vi "Assignment #3 - Sarah Bailey.vi"() -> ()   [LabVIEW 2013]
panel:
  out "Calculated Tolerance":dbl
  out "ROOT":dbl
  in  "Tolerance":dbl min=0.0
  in  "XHI":dbl=1e-16 min=1e-16
  in  "XLO":dbl=1e-16 min=1e-16
  # "Developed by: Sarah Bailey\nEngineering Applications Lab\nAssignment #3\nProfessor Wellin\nWorked with: Clair Cummingham and Alex Offredi"
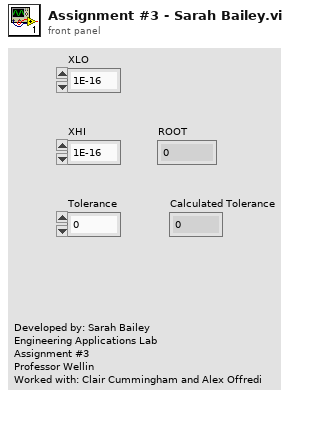
[diagram p1: front panel]
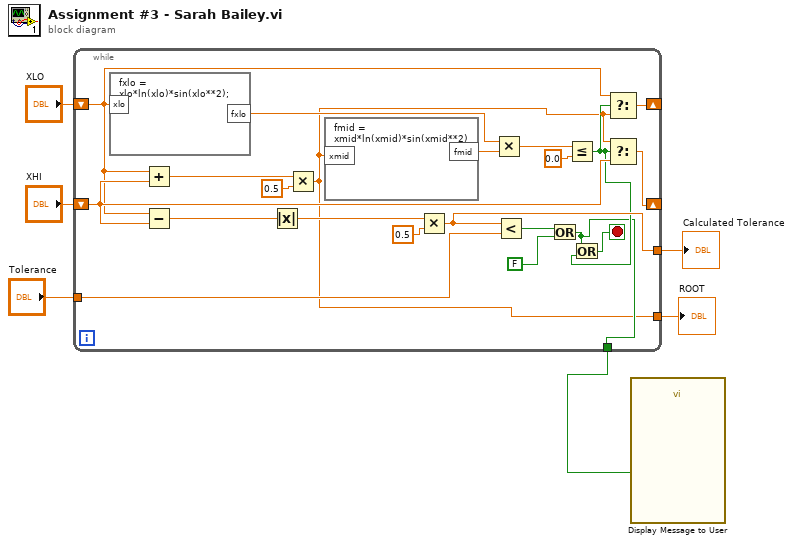
[diagram p0: block diagram]
diagram:
  n1 = while {
    shift-right: [w22] -> _
    shift-left: "XLO" -> [w16]
    shift-right: [w23] -> _
    shift-left: "XHI" -> [w21]
    tunnel: [w7] -> w4
    tunnel: [w8] -> w3
    tunnel: "Tolerance" -> [w12]
    tunnel: [w11] -> w1
    stop <- w9 stop-if-true
    n2 = formula code="fxlo = xlo*ln(xlo)*sin(xlo**2);"("xlo"=w16) -> ("fxlo"=w15:dbl)
    n3 = Add(x=w16, y=w21) -> (x+y=w27:dbl)
    n4 = Subtract(x=w16, y=w21) -> (x-y=w20:dbl)
    n5 = Absolute Value(x=w20) -> (abs(x)=w19:dbl)
    n6 = Multiply(x=w27, y=0.5) -> (x*y=w7:dbl)
    n7 = formula code="fmid = xmid*ln(xmid)*sin(xmid**2) ;"("xmid"=w7) -> ("fmid"=w14:dbl)
    n8 = Multiply(x=w19, y=0.5) -> (x*y=w11:dbl)
    n9 = Multiply(x=w15, y=w14) -> (x*y=w25:dbl)
    n10 = Less?(x=w11, y=w12) -> (x < y?=w17:bool)
    n11 = Or(x=w17, y=FALSE) -> (x .or. y?=w8:bool)
    n12 = Less Or Equal?(x=w25, y=0.0) -> (x <= y?=w10:bool)
    n13 = Or(x=w8, y=w10) -> (x .or. y?=w9:bool)
    n14 = Select(t=w16, s=w10, f=w7) -> (s? t:f=w22:dbl)
    n15 = Select(t=w7, s=w10, f=w21) -> (s? t:f=w23:dbl)
  }
  "ROOT" <- w4
  "Calculated Tolerance" <- w1
  n16 = call "Display Message to User"("Enable"=w3) -> ()  [unwired: 9 in, 2 out]
